vi "文本文件（读取文本文件函数）.vi"() -> ()   [LabVIEW 2017]
panel:
  out "文本":string
  out "波形图":dbl[](graph)
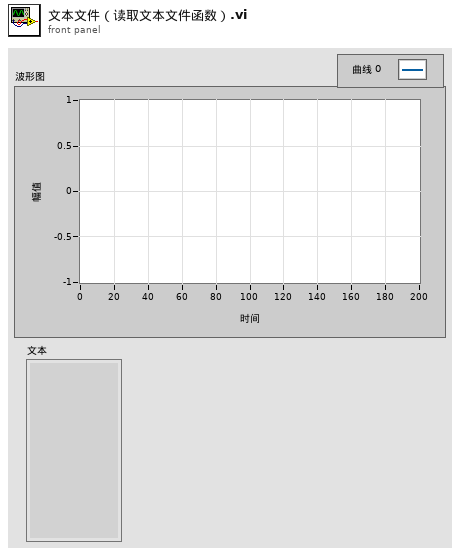
[diagram p1: front panel]
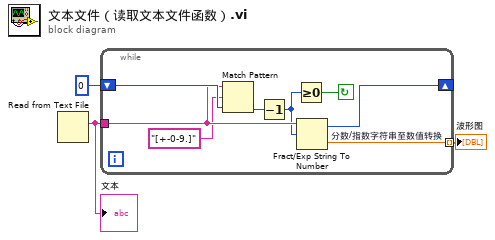
[diagram p0: block diagram]
diagram:
  n1 = Read from Text File() -> (text=w2:string)  [unwired: 4 in, 3 out]
  "文本" <- w2
  n2 = while {
    shift-right: [w8] -> _
    shift-left: 0 -> [w11]
    tunnel: w2 -> [w9]
    tunnel: [w7] -> w1 mode=indexing
    stop <- w10 continue-if-true
    n3 = Match Pattern(string=w9, regular expression="[+-0-9.]" ("正则表达式"), offset (0)=w11) -> (offset past match=w4:i32)  [unwired: 3 out]
    n4 = Decrement(x=w4) -> (x-1=w5:i32)
    n5 = Greater Or Equal To 0?(x=w5) -> (x >= 0?=w10:bool)
    n6 = Fract/Exp String To Number "分数/指数字符串至数值转换"(string=w9, offset=w5) -> (offset past number=w8:i32, number=w7:dbl)  [unwired: 2 in]
  }
  "波形图" <- w1
